vi "updateSettlingInfo.vi"(8 "error in (no error)":errorcluster, 11 "Model in":refnum<class "Model.lvclass">) -> (0 "error out":errorcluster, 3 "Model out":refnum<class "Model.lvclass">)   [LabVIEW 2015, in "Model.lvclass"]
uses:
  Model.lvclass
  Model.lvclass/Model.ctl
  <userlib>/Common/Devices/DistanceGauge/DistanceGauge/DistanceGauge.lvclass/DistanceGauge.ctl
  ApplicationElements/SystemController/SystemController.lvclass
  <userlib>/Common/Devices/DistanceGauge/DistanceGauge/DistanceGauge.lvclass
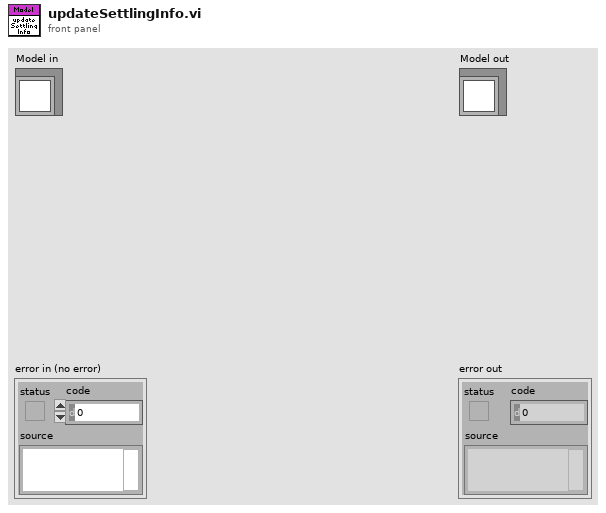
[diagram p1: front panel]
types:
  T1 = typedef "DistanceGauge.lvlib/Distance Data.ctl" = cluster{"Distance Measured":dbl[unit]}
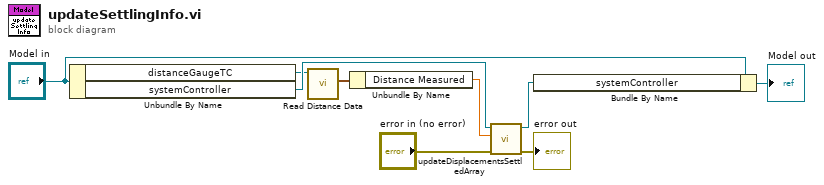
[diagram p0: block diagram]
diagram:
  n1 = Unbundle By Name("Model in") -> ("distanceGaugeTC"=w5:refnum<class "DistanceGaugeTC.lvclass">, "systemController"=w8:refnum<class "SystemController.lvclass">)
  n2 = call <userlib>:"Read Distance Data.vi"("DistanceGauge in"=w5) -> ("Distance Data"=w4:T1)  [unwired: 9 in, 1 out]
  n3 = Unbundle By Name(w4) -> ("Distance Measured"=w3:dbl[unit])
  n4 = call "updateDisplacementsSettledArray.vi"("error in (no error)"="error in (no error)", "Distance Measured"=w3, "SystemController in"=w8) -> ("error out"=→"error out":errorcluster, "SystemController out"=w7:refnum<class "SystemController.lvclass">)  [unwired: 6 in, 1 out]
  n5 = Bundle By Name(cluster="Model in", "systemController"=w7) -> (→"Model out":refnum<class "Model.lvclass">)
